vi "NIDAQmx Logic.vi"(8 "error in (no error)":errorcluster, 10 "Measurement Configuration":T2, 11 "Session Factory in":refnum<class "Session Factory.lvclass">) -> (0 "error out":errorcluster, 3 "Measurement Results":T1)   [LabVIEW 2021, in "NIDAQmxMeasurement.lvlib"]
doc: "This VI performs the DAQmx measurement."
uses:
  NIDAQmxMeasurement.lvlib
  Measurement Configuration.ctl
  Measurement Results.ctl
  Source/NI DAQmx/Session/Session Factory/Session Factory.lvclass
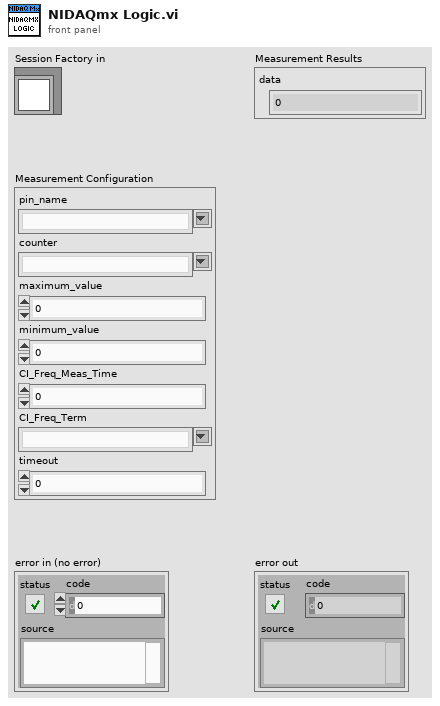
[diagram p1: front panel]
types:
  T1 = typedef "NIDAQmxMeasurement.lvlib/Measurement Results.ctl" = cluster{"data":dbl}
  T2 = typedef "NIDAQmxMeasurement.lvlib/Measurement Configuration.ctl" = cluster{"pin_name":string, "counter":string, "maximum_value":dbl, "minimum_value":dbl, "CI_Freq_Meas_Time":dbl, "CI_Freq_Term":string, "timeout":dbl}
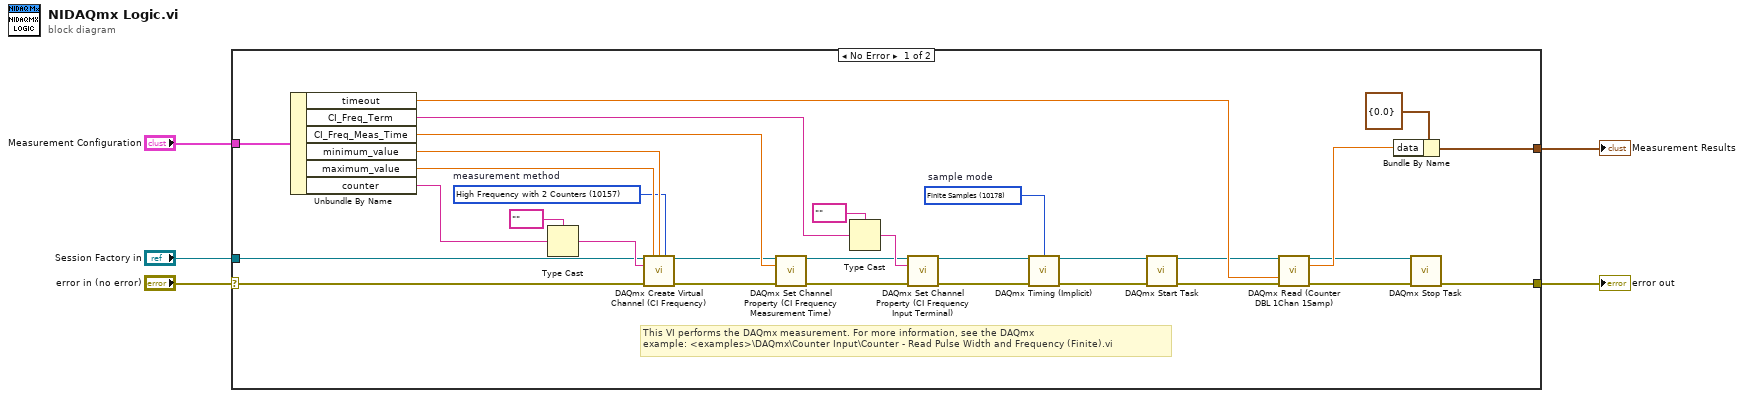
[diagram p0: block diagram]
diagram:
  n1 = case shown="No Error" "error in (no error)" {
    selector: "error in (no error)" -> [w6 w37]
    tunnel: "Measurement Configuration" -> [w36 _]
    tunnel: [w35 _] -> w4
    tunnel: [w16 w37] -> w3
    tunnel: "Session Factory in" -> [w7 _]
    frame No Error {
      w17 = 10157 items=["Low Frequency with 1 Counter"=10105, "High Frequency with 2 Counters"=10157, "Large Range with 2 Counters"=10205, "Dynamic Averaging"=16065]  # measurement method
      w22 = 10178 items=["Finite Samples"=10178, "Continuous Samples"=10123, "Hardware Timed Single Point"=12522]  # sample mode
      # "This VI performs the DAQmx measurement. For more information, see the DAQmx \nexample: <examples>\\DAQmx\\Counter Input\\Counter - Read Pulse Width and Frequency (Finite).vi"
      n2 = Unbundle By Name(w36) -> ("timeout"=w32:dbl, "CI_Freq_Term"=w31:string, "CI_Freq_Meas_Time"=w28:dbl, "minimum_value"=w23:dbl, "maximum_value"=w24:dbl, "counter"=w27:string)
      n3 = Type Cast(type=tag "" ("counter"), x=w27) -> (*(type *) &x=w26:tag)
      n4 = call "DAQmx Create Virtual Channel (CI Frequency).vi"("task in"=w7, "maximum value"=w24, "minimum value"=w23, "measurement method"=w17, "counter"=w26, "error in"=w6) -> ("task out"=w10:refnum<class "Session Factory.lvclass">, "error out"=w8:errorcluster)  [unwired: 8 in]
      n5 = call "DAQmx Set Channel Property (CI Frequency Measurement Time).vi"("task in"=w10, "CI.Freq.MeasTime"=w28, "error in"=w8) -> ("task out"=w11:refnum<class "Session Factory.lvclass">, "error out"=w9:errorcluster)  [unwired: 11 in]
      n6 = Type Cast(type=tag "" ("CI.Freq.Term"), x=w31) -> (*(type *) &x=w30:tag)
      n7 = call "DAQmx Set Channel Property (CI Frequency Input Terminal).vi"("task in"=w11, "CI.Freq.Term"=w30, "error in"=w9) -> ("task out"=w20:refnum<class "Session Factory.lvclass">, "error out"=w18:errorcluster)  [unwired: 11 in]
      n8 = call "DAQmx Timing (Implicit).vi"("task in"=w20, "sample mode"=w22, "error in"=w18) -> ("task out"=w21:refnum<class "Session Factory.lvclass">, "error out"=w19:errorcluster)  [unwired: 11 in]
      n9 = call "DAQmx Start Task.vi"("task in"=w21, "error in"=w19) -> ("task out"=w14:refnum<class "Session Factory.lvclass">, "error out"=w12:errorcluster)  [unwired: 12 in]
      n10 = call "DAQmx Read (Counter DBL 1Chan 1Samp).vi"("task in"=w14, "timeout"=w32, "error in"=w12) -> ("task out"=w15:refnum<class "Session Factory.lvclass">, "data"=w34:dbl, "error out"=w13:errorcluster)  [unwired: 10 in]
      n11 = Bundle By Name(cluster=T1 {"data"=0.0} ("Measurement Results"), "data"=w34) -> (w35:T1)
      n12 = call "DAQmx Stop Task.vi"("task in"=w15, "error in"=w13) -> ("error out"=w16:errorcluster)  [unwired: 12 in, 1 out]
    }
    frame Error {
    }
  }
  "Measurement Results" <- w4
  "error out" <- w3
